vi "Get Theme Data.vi"(8 "error in":errorcluster, 11 "VI Refnum":refnum<vi>) -> (0 "error out":errorcluster, 1 "Theme":u16(ring)=3 items=["Light Theme", "Light Medium Contrast", "Light High Contrast", "Dark Theme", "Dark Medium Contrast", "Dark High Constrast"], 2 "Theme Path":path, 3 "VI Refnum out":refnum<vi>, 4 "Found?":bool)   [LabVIEW 2021, in "Material SubVIs.lvlib"]
doc: "Get the VI's user tag data if it exists for the last theme and last theme level applied.\n\n<b>Code Developed By:</b> +\nDaniel Coons +\nTechnology Service Corporation +\nwww.tsc.com/atcs"
uses:
  Material SubVIs.lvlib
  <vilib>/UserTags/UserTags.lvlib
  <vilib>/AppBuilder/AB_Relative_Path_Type.ctl
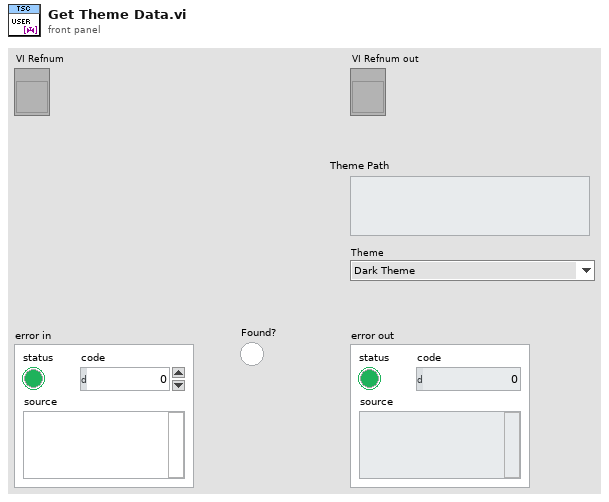
[diagram p1: front panel]
types:
  T1 = typedef "AB_Relative_Path_Type.ctl" = enum16{"<none>", "relativeToCommon", "relativeToAppDir", "relativeToProject"}
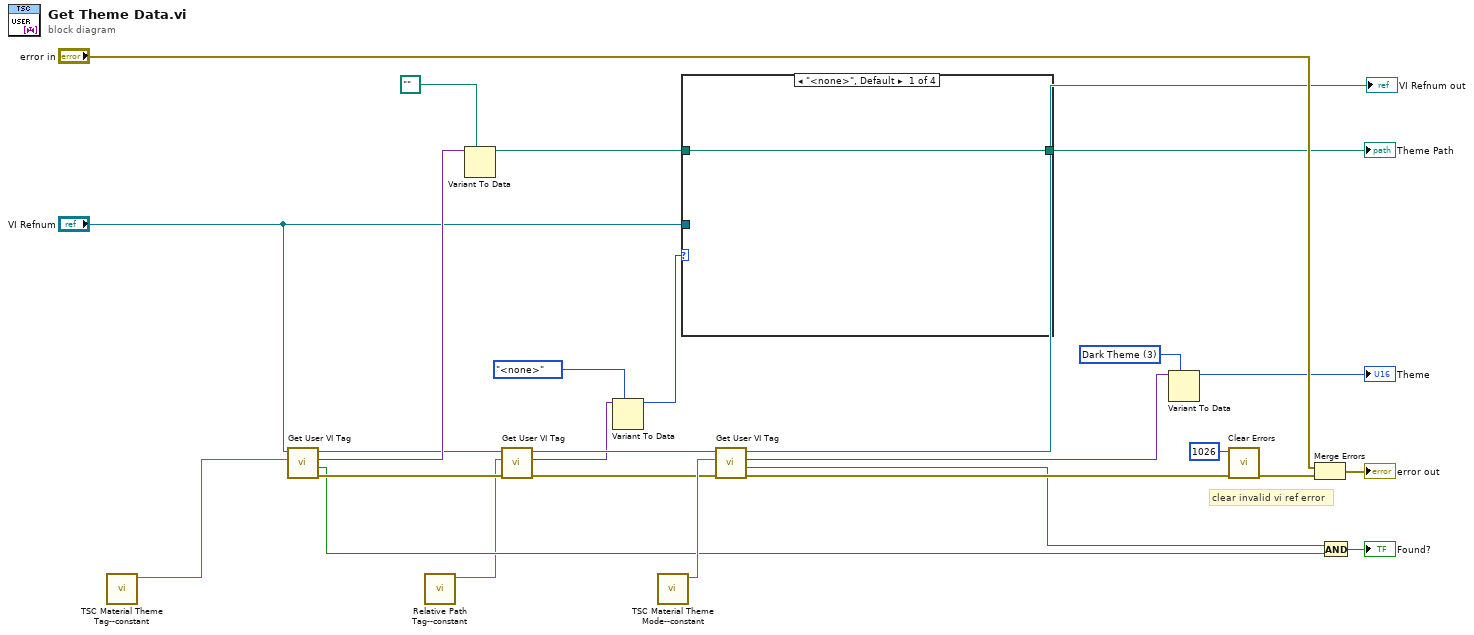
[diagram p0: block diagram]
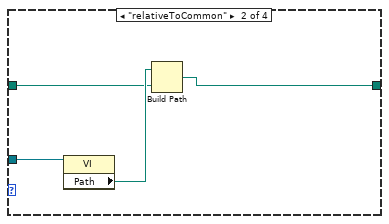
[diagram p2: hidden frame]
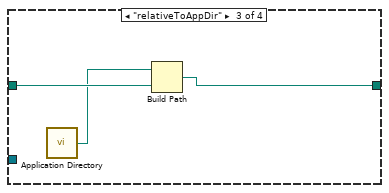
[diagram p3: hidden frame]
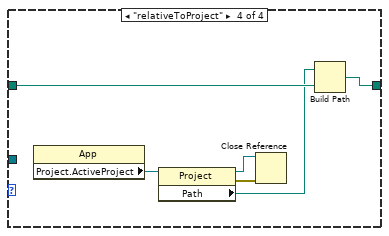
[diagram p4: hidden frame]
diagram:
  w17 = u16 3 items=["Light Theme", "Light Medium Contrast", "Light High Contrast", "Dark Theme", "Dark Medium Contrast", "Dark High Constrast"] ("Theme")
  # "clear invalid vi ref error"
  n1 = call "TSC Material Theme Tag--constant.vi"() -> ("Theme Path Tag"=w22:string)  [unwired: 11 in]
  n2 = call <vilib>:"Get User VI Tag.vi"("Tag Name"=w22, "VI Refnum"="VI Refnum") -> ("error out"=w27:errorcluster, "Was Tag Found?"=w14:bool, "Value"=w20:variant, "dup VI Refnum"=w9:refnum<vi>)  [unwired: 6 in]
  n3 = call "Relative Path Tag--constant.vi"() -> ("Relative Path Tag"=w7:string)  [unwired: 11 in]
  n4 = Variant To Data(type=path "", Variant=w20) -> (data=w3:path)  [unwired: 1 in, 1 out]
  n5 = call <vilib>:"Get User VI Tag.vi"("error in (no error)"=w27, "Tag Name"=w7, "VI Refnum"=w9) -> ("error out"=w10:errorcluster, "Value"=w6:variant, "dup VI Refnum"=w8:refnum<vi>)  [unwired: 5 in, 1 out]
  n6 = Variant To Data(type=AB_Relative_Path_Type."<none>" ("relativeType"), Variant=w6) -> (data=w4:T1)  [unwired: 1 in, 1 out]
  n7 = call "TSC Material Theme Mode--constant.vi"() -> ("Theme Path Tag"=w21:string)  [unwired: 11 in]
  n8 = case shown="\"<none>\", Default" w4 {
    tunnel: w3 -> [w28 w30 w35 w41]
    tunnel: "VI Refnum" -> [_ w32 _ _]
    tunnel: [w28 w29 w34 w40] -> w1
    frame "<none>", Default {
    }
    frame "relativeToCommon" {
      n9 = property class="VI"(reference=w32) -> ("Path"=w31:path)  [unwired: 1 in, 2 out]
      n10 = Build Path(base path=w31, name or relative path=w30) -> (appended path=w29:path)
    }
    frame "relativeToAppDir" {
      n11 = call <vilib>:"Application Directory.vi"() -> ("Application Directory"=w33:path)
      n12 = Build Path(base path=w33, name or relative path=w35) -> (appended path=w34:path)
    }
    frame "relativeToProject" {
      n13 = property class="App"() -> ("Project.ActiveProject"=w39:refnum<vi>)  [unwired: 2 in, 2 out]
      n14 = property class="Project"(reference=w39) -> (reference out=w36:refnum<vi>, error out=w37:errorcluster, "Path"=w38:path)  [unwired: 1 in]
      n15 = Close Reference(reference=w36, error in (no error)=w37) -> ()  [unwired: 1 out]
      n16 = Build Path(base path=w38, name or relative path=w41) -> (appended path=w40:path)
    }
  }
  "Theme Path" <- w1
  n17 = call <vilib>:"Get User VI Tag.vi"("error in (no error)"=w10, "Tag Name"=w21, "VI Refnum"=w8) -> ("error out"=w26:errorcluster, "Was Tag Found?"=w13:bool, "Value"=w18:variant, "dup VI Refnum"=→"VI Refnum out":refnum<vi>)  [unwired: 5 in]
  n18 = Variant To Data(type=w17, Variant=w18) -> (data=→"Theme":u16)  [unwired: 1 in, 1 out]
  n19 = call <vilib>:"Clear Errors.vi"("error in (no error)"=w26, "specific error code to clear (0: all)"=1026) -> ("error out"=w23:errorcluster)  [unwired: 4 in, 1 out]
  n20 = Merge Errors("error in", w23) -> (→"error out":errorcluster)
  n21 = And(x=w13, y=w14) -> (x .and. y?=→"Found?":bool)
